vi "series.get.vi"() -> ()   [LabVIEW 2024]
uses:
  <vilib>/httpClient/POSTBuffer.vi
  <vilib>/httpClient/LabVIEWHTTPClient.lvlib
panel:
  out "prev_seriesID":i32
  out "seriesID":i32
  in  "url":string="https://www.comics.org/series/184161/"
  out "body":string
  out "error out":errorcluster
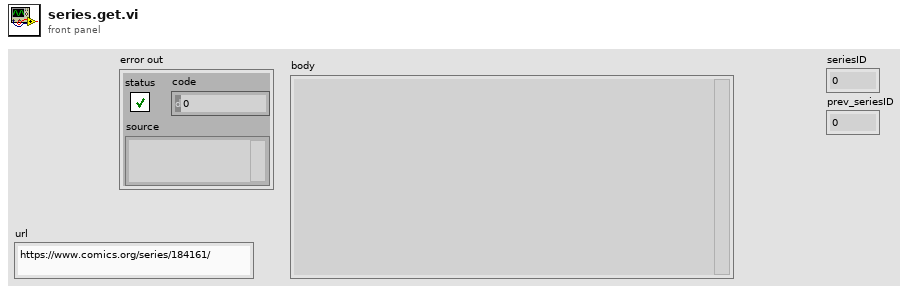
[diagram p1: front panel]
types:
  T1 = typedef "LabVIEWHTTPClient.lvlib/ClientHandle.ctl" = refnum<k1>
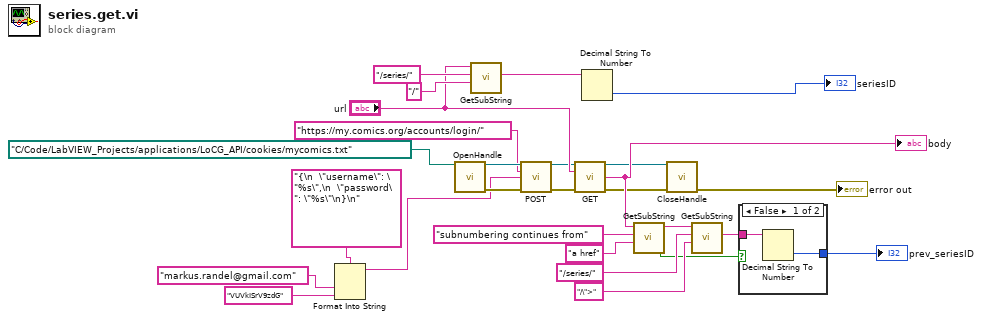
[diagram p0: block diagram]
diagram:
  n1 = Format Into String(format string="{\n  \"username\": \"%s\",\n  \"password\": \"%s\"\n}\n", "markus.randel@gmail.com", "VUVkISrV9zdG") -> (resulting string=w1:string)  [unwired: 2 in, 1 out]
  n2 = call <vilib>:"OpenHandle.vi"("cookie file"=path "C:/Code/LabVIEW_Projects/applications/LoCG_API/cookies/mycomics.txt") -> ("client handle out"=w7:T1, "error out"=w6:errorcluster)  [unwired: 13 in]
  n3 = call "GetSubString.vi"("End Search"="/" ("regular expression"), "Start Search"="/series/" ("regular expression"), "String In"="url") -> ("Match"=w25:string)  [unwired: 6 in, 2 out]
  n4 = call-poly <vilib>:"POST.vi"("client handle"=w7, "url"="https://my.comics.org/accounts/login/", "buffer"=w1, "error in (no error)"=w6) -> ("client handle out"=w9:T1, "error out"=w8:errorcluster)  [unwired: 8 in, 2 out]
  n5 = call <vilib>:"GET.vi"("client handle"=w9, "url"="url", "error in (no error)"=w8) -> ("client handle out"=w10:T1, "body"=w23:string, "error out"=w12:errorcluster)  [unwired: 9 in, 1 out]
  "body" <- w23
  n6 = Decimal String To Number(string=w25) -> (number=→"seriesID":i32)  [unwired: 2 in, 1 out]
  n7 = call "GetSubString.vi"("End Search"="a href", "Start Search"="subnumbering continues from", "String In"=w23) -> ("Not Found?"=w16:bool, "Following String Out"=w20:string)  [unwired: 6 in, 1 out]
  n8 = call <vilib>:"CloseHandle.vi"("client handle"=w10, "error in (no error)"=w12) -> ("error out"=→"error out":errorcluster)  [unwired: 13 in]
  n9 = call "GetSubString.vi"("End Search"="/\">" ("Start Search"), "Start Search"="/series/", "String In"=w20) -> ("Match"=w17:string)  [unwired: 6 in, 2 out]
  n10 = case shown="False" w16 {
    tunnel: w17 -> [w29 _]
    tunnel: [w28 _] -> w15
    frame False {
      n11 = Decimal String To Number(string=w29) -> (number=w28:i32)  [unwired: 2 in, 1 out]
    }
    frame True {
    }
  }
  "prev_seriesID" <- w15
